vi "Fetch Package Details.vi"(8 "error in (no error)":errorcluster, 9 "Package Version":string, 10 "Package Name":string, 11 "HTTP handle in":T1) -> (0 "error out":errorcluster, 2 "Pkg Version":refnum<class "Package Version.lvclass">, 3 "HTTP handle out":T1)   [LabVIEW 2016, in "Packages.lvlib" / "GPM.lvlib"]
uses:
  GPM.lvlib
  Package Version_class/Package Version.lvclass
  <vilib>/httpClient/ClientHandle.ctl
  Package Version_class/Package Version.lvclass/Package Version.ctl
  <vilib>/addons/JSON API/JSON Value/Set from JSON string.vi
  Package Version_class/Write Version.vi
  Package Version_class/Write ReleaseDate.vi
  Package Version_class/Write Vendor.vi
  Package Version_class/Write IconURL.vi
  Package Version_class/Write DisplayName.vi
  Package Version_class/Write Description.vi
  Package Version_class/Write PackageURL.vi
  Package Version_class/Write Author.vi
  Package Version_class/Write Release Notes.vi
  Package Version_class/Write Dependencies.vi
  <vilib>/addons/JSON API/JSON Object/Get Object.vi
  <vilib>/addons/JSON API/JSON Value/JSON Value.lvclass
  <vilib>/httpClient/LabVIEWHTTPClient.lvlib
  <vilib>/addons/JSON API/Get Polymorphic/JSON GetSet.lvlib
  <vilib>/addons/JSON API/JSON Scalar/JSON Scalar.lvclass
  WSsupport/WSsupport.lvlib
  <vilib>/addons/JSON API/JSON Object/JSON Object.lvclass
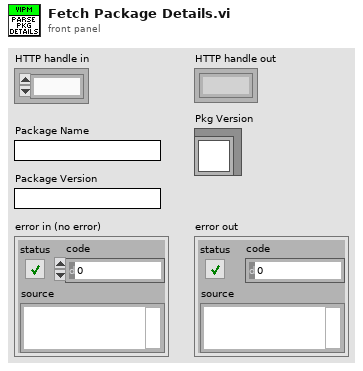
[diagram p1: front panel]
types:
  T1 = typedef "LabVIEWHTTPClient.lvlib/ClientHandle.ctl" = refnum<k1>
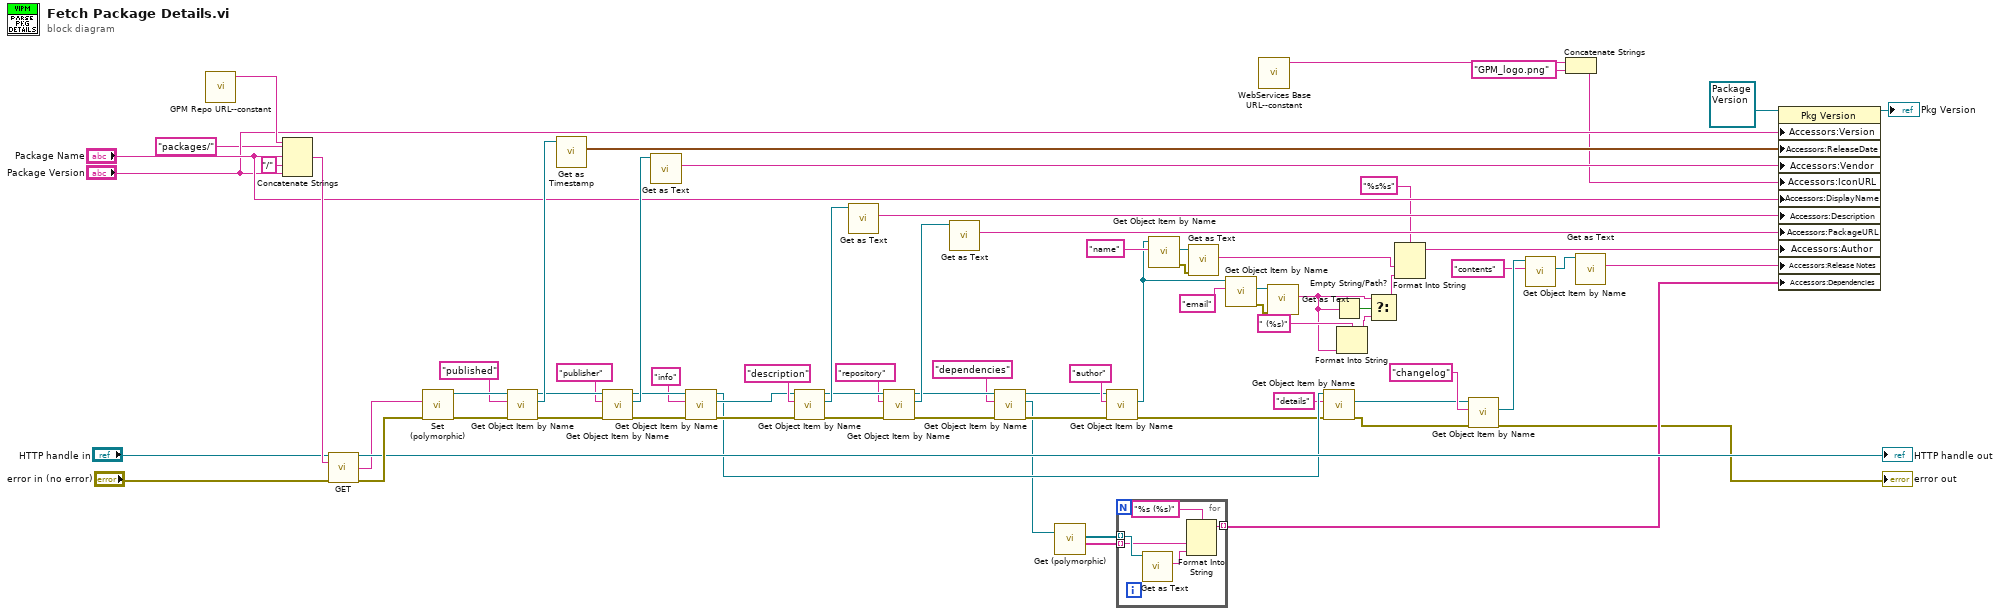
[diagram p0: block diagram]
diagram:
  n1 = call "GPM Repo URL--constant.vi"() -> ("GPM Repo URL"=w72:string)  [unwired: 11 in]
  n2 = Concatenate Strings(w72, "packages/" ("string"), "Package Name", "/" ("string"), "Package Version") -> (w69:string)
  n3 = call <vilib>:"GET.vi"("client handle"="HTTP handle in", "url"=w69, "error in (no error)"="error in (no error)") -> ("client handle out"=→"HTTP handle out":T1, "body"=w65:string, "error out"=w70:errorcluster)  [unwired: 9 in, 1 out]
  n4 = call-poly <vilib>:"Set (polymorphic).vi"("error in (no error)"=w70, "JSON stream"=w65) -> ("error out"=w66:errorcluster, "JSON Value out"=w63:refnum<class "JSON Value.lvclass">)  [unwired: 7 in, 1 out]
  n5 = call <vilib>:"Get Object Item by Name.vi"("error in (no error)"=w66, "name"="published", "JSON Value In"=w63) -> ("error out"=w64:errorcluster, "Value"=w61:refnum<class "JSON Value.lvclass">, "JSON Value Out"=w58:refnum<class "JSON Value.lvclass">)  [unwired: 5 in, 1 out]
  n6 = call <vilib>:"Get as Timestamp.vi"("JSON Value in"=w61) -> ("Time Stamp"=w60:timestamp)  [unwired: 8 in, 2 out]
  n7 = call <vilib>:"Get Object Item by Name.vi"("error in (no error)"=w64, "name"="publisher", "JSON Value In"=w58) -> ("error out"=w59:errorcluster, "Value"=w56:refnum<class "JSON Value.lvclass">, "JSON Value Out"=w20:refnum<class "JSON Value.lvclass">)  [unwired: 5 in, 1 out]
  n8 = call <vilib>:"Get as Text.vi"("JSON Scalar in"=w56) -> ("LabVIEW Text"=w55:string)  [unwired: 8 in, 2 out]
  n9 = call <vilib>:"Get Object Item by Name.vi"("error in (no error)"=w59, "name"="info", "JSON Value In"=w20) -> ("error out"=w21:errorcluster, "Value"=w18:refnum<class "JSON Value.lvclass">, "JSON Value Out"=w17:refnum<class "JSON Value.lvclass">)  [unwired: 5 in, 1 out]
  n10 = call <vilib>:"Get Object Item by Name.vi"("error in (no error)"=w21, "name"="description", "JSON Value In"=w18) -> ("error out"=w53:errorcluster, "Value"=w51:refnum<class "JSON Value.lvclass">, "JSON Value Out"=w48:refnum<class "JSON Value.lvclass">)  [unwired: 5 in, 1 out]
  n11 = call <vilib>:"Get as Text.vi"("JSON Scalar in"=w51) -> ("LabVIEW Text"=w50:string)  [unwired: 8 in, 2 out]
  n12 = call <vilib>:"Get Object Item by Name.vi"("error in (no error)"=w53, "name"="repository", "JSON Value In"=w48) -> ("error out"=w49:errorcluster, "Value"=w46:refnum<class "JSON Value.lvclass">, "JSON Value Out"=w13:refnum<class "JSON Value.lvclass">)  [unwired: 5 in, 1 out]
  n13 = call <vilib>:"Get as Text.vi"("JSON Scalar in"=w46) -> ("LabVIEW Text"=w45:string)  [unwired: 8 in, 2 out]
  n14 = call <vilib>:"Get Object Item by Name.vi"("error in (no error)"=w49, "name"="dependencies", "JSON Value In"=w13) -> ("error out"=w14:errorcluster, "Value"=w8:refnum<class "JSON Value.lvclass">, "JSON Value Out"=w12:refnum<class "JSON Value.lvclass">)  [unwired: 5 in, 1 out]
  n15 = call-poly <vilib>:"Get (polymorphic).vi"("JSON Object in"=w8) -> ("Sub-Item Names"=w7:string[], "Sub-Items"=w6:refnum<class "JSON Value.lvclass">[])  [unwired: 7 in, 2 out]
  n16 = call <vilib>:"Get Object Item by Name.vi"("error in (no error)"=w14, "name"="author", "JSON Value In"=w12) -> ("error out"=w9:errorcluster, "Value"=w10:refnum<class "JSON Value.lvclass">)  [unwired: 5 in, 2 out]
  n17 = for {
    tunnel: w7 -> [w79] mode=indexing
    tunnel: w6 -> [w80] mode=indexing
    tunnel: [w76] -> w5 mode=indexing
    n18 = call <vilib>:"Get as Text.vi"("JSON Scalar in"=w80) -> ("LabVIEW Text"=w78:string)  [unwired: 8 in, 2 out]
    n19 = Format Into String(format string="%s (%s)", w79, w78) -> (resulting string=w76:string)  [unwired: 2 in, 1 out]
  }
  n20 = call <vilib>:"Get Object Item by Name.vi"("name"="name", "JSON Value In"=w10) -> ("error out"=w4:errorcluster, "Value"=w41:refnum<class "JSON Value.lvclass">)  [unwired: 6 in, 2 out]
  n21 = call <vilib>:"Get as Text.vi"("error in (no error)"=w4, "JSON Scalar in"=w41) -> ("LabVIEW Text"=w27:string)  [unwired: 7 in, 2 out]
  n22 = call <vilib>:"Get Object Item by Name.vi"("name"="email", "JSON Value In"=w10) -> ("error out"=w3:errorcluster, "Value"=w40:refnum<class "JSON Value.lvclass">)  [unwired: 6 in, 2 out]
  n23 = call "WebServices Base URL--constant.vi"() -> ("WebServices Base URL"=w31:string)  [unwired: 11 in]
  n24 = call <vilib>:"Get as Text.vi"("error in (no error)"=w3, "JSON Scalar in"=w40) -> ("LabVIEW Text"=w23:string)  [unwired: 7 in, 2 out]
  n25 = call <vilib>:"Get Object Item by Name.vi"("error in (no error)"=w9, "name"="details", "JSON Value In"=w17) -> ("error out"=w2:errorcluster, "Value"=w15:refnum<class "JSON Value.lvclass">)  [unwired: 5 in, 2 out]
  n26 = Empty String/Path?(string/path=w23) -> (empty?=w26:bool)
  n27 = Format Into String(format string=" (%s)", w23) -> (resulting string=w24:string)  [unwired: 2 in, 1 out]
  n28 = Select(t=w23, s=w26, f=w24) -> (s? t:f=w22:string)
  n29 = Format Into String(format string="%s%s", w27, w22) -> (resulting string=w39:string)  [unwired: 2 in, 1 out]
  n30 = call <vilib>:"Get Object Item by Name.vi"("error in (no error)"=w2, "name"="changelog", "JSON Value In"=w15) -> ("error out"=→"error out":errorcluster, "Value"=w36:refnum<class "JSON Value.lvclass">)  [unwired: 5 in, 2 out]
  n31 = call <vilib>:"Get Object Item by Name.vi"("name"="contents", "JSON Value In"=w36) -> ("Value"=w34:refnum<class "JSON Value.lvclass">)  [unwired: 6 in, 3 out]
  n32 = Concatenate Strings(w31, "GPM_logo.png" ("string")) -> (w29:string)
  n33 = call <vilib>:"Get as Text.vi"("JSON Scalar in"=w34) -> ("LabVIEW Text"=w33:string)  [unwired: 8 in, 2 out]
  n34 = property class="Pkg Version"(reference=refnum<class "Package Version.lvclass"> refnum ("Packages.lvlib:Pkg Version"), "Accessors:Version"="Package Version", "Accessors:ReleaseDate"=w60, "Accessors:Vendor"=w55, "Accessors:IconURL"=w29, "Accessors:DisplayName"="Package Name", "Accessors:Description"=w50, "Accessors:PackageURL"=w45, "Accessors:Author"=w39, "Accessors:Release Notes"=w33, "Accessors:Dependencies"=w5) -> (reference out=→"Pkg Version":refnum<class "Package Version.lvclass">)  [unwired: 1 in, 1 out]
